vi "1Dto2D - Copy.vi"(11 "Array":dbl[](array[numeric])) -> (3 "output array":dbl[][](array[numeric]))   [LabVIEW 2014]
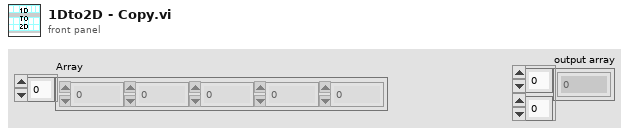
[diagram p1: front panel]
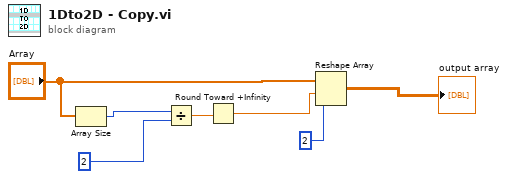
[diagram p0: block diagram]
diagram:
  n1 = Array Size(array="Array") -> (size(s)=w5:i32)
  n2 = Divide(x=w5, y=2 ("x")) -> (x/y=w3:dbl)
  n3 = Round Toward +Infinity(x=w3) -> (ceil(x): smallest int >= x=w2:dbl)
  n4 = Reshape Array("Array", w2, 2 ("dimension size")) -> (→"output array":dbl[][])
